vi "Inputs.vi"(8 "error in (no error)":errorcluster, 11 "State in":T1={"State"=enum."Idle", "Start Time"=timestamp(0 s since 1904-01-01), "Configuration"={"Cycle Period"=0.0, "Bronkhorst M13"={"VISA resource name"="", "Simulated?"=FALSE}, "Flow Meter Type"="", "Bronkhorst M14"={"VISA resource name"="", "Simulated?"=FALSE}}, "Current Time"=timestamp(0 s since 1904-01-01), "First Iteration"=FALSE, "Data"={"Flow Meter Read(g/min)"=0.0, "Density"=0.0, "Temp (C)"=0.0}, "Process Name"="", "Log Started"=FALSE}) -> (0 "error out":errorcluster, 3 "State out":T1={"State"=enum."Idle", "Start Time"=timestamp(0 s since 1904-01-01), "Configuration"={"Cycle Period"=0.0, "Bronkhorst M13"={"VISA resource name"="", "Simulated?"=FALSE}, "Flow Meter Type"="", "Bronkhorst M14"={"VISA resource name"="", "Simulated?"=FALSE}}, "Current Time"=timestamp(0 s since 1904-01-01), "First Iteration"=FALSE, "Data"={"Flow Meter Read(g/min)"=0.0, "Density"=0.0, "Temp (C)"=0.0}, "Process Name"="", "Log Started"=FALSE})   [LabVIEW 2018, in "Flow Module.lvlib" / "Flow Module Engine.lvlib"]
uses:
  Flow Module Engine.lvlib
  State Cluster.ctl
  State Enum.ctl
  Feed Module/Controls/Flow Module Settings Cluster.ctl
  Mettler Toledo/Controls/Settings Cluster.ctl
  Tag VIs/Tag FGV Operation Enum.ctl
  Bronkhorst M13 Flow Meter/Bronkhorst M13 Flow Meter.lvlib
  Bronkhorst M14 Flow Meter/Bronkhorst M14 Flow Meter.lvlib
  Shared Variables/Dynamic Shared Variables.lvlib
  Flow Module.lvlib
  Mettler Toledo/Mettler Toledo.lvlib
panel:
  # "Flow Meter Settings"
  # "Flow Meter Settings"
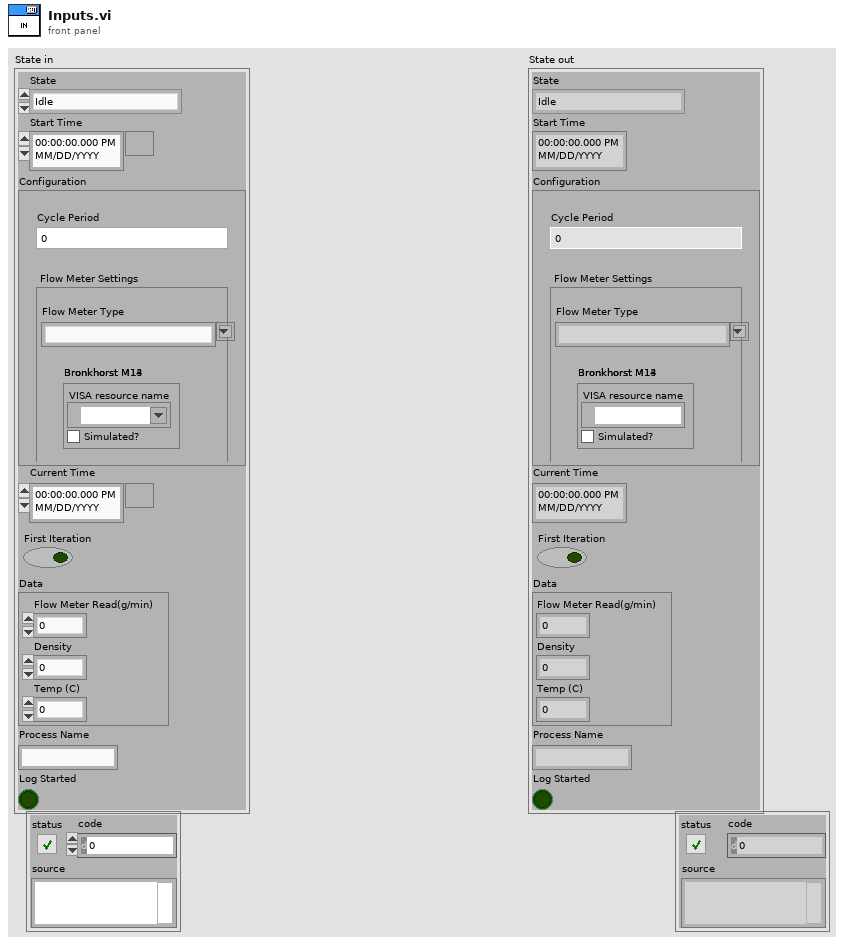
[diagram p1: front panel]
types:
  T1 = typedef "Flow Module.lvlib/Flow Module Engine.lvlib/State Cluster.ctl" = cluster{"State":T2, "Start Time":timestamp, "Configuration":T3, "Current Time":timestamp, "First Iteration":bool, "Data":cluster{"Flow Meter Read(g/min)":dbl, "Density":dbl, "Temp (C)":dbl}, "Process Name":string, "Log Started":bool}
  T2 = typedef "Flow Module.lvlib/Flow Module Engine.lvlib/State Enum.ctl" = enum16{"Measuring", "Idle"}
  T3 = typedef "Flow Module.lvlib/Flow Module Settings Cluster.ctl" = cluster{"Cycle Period":dbl, "Bronkhorst M13":T4, "Flow Meter Type":string, "Bronkhorst M14":T4}
  T4 = typedef "Mettler Toledo.lvlib/Settings Cluster.ctl" = cluster{"VISA resource name":refnum<visa-resource-name>, "Simulated?":bool}
  T5 = typedef "Tag FGV Operation Enum.ctl" = enum16{"Init", "Set Notification Queue", "Create Tag", "Commit", "Write Tag (Numeric)", "Write Tag (Boolean)", "Read All Tags", "Read One Tag", "Delete Tag Category", "Set Alarm Parameters (Numeric)", "Set Alarm Parameters (Boolean)", "Enable All Alarms", "Disable All Alarms", "Delete All Tags", "Read Alarms", "Ack Alarm", "Read Alarm Parameters (Numeric)", "Read Alarm Parameters (Boolean)"}
  T6 = typedef "Bronkhorst M13 Flow Meter.lvlib/Settings Cluster.ctl" = cluster{"VISA resource name":refnum<visa-resource-name>, "Simulated?":bool}
  T7 = typedef "Bronkhorst M14 Flow Meter.lvlib/Settings Cluster.ctl" = cluster{"VISA resource name":refnum<visa-resource-name>, "Simulated?":bool}
  T8 = typedef "Flow Module.lvlib/Tag Cluster.ctl" = cluster{"Flow Tag":string, "Input Disconnected":string, "Density Tag":string, "Temp Tag":string}
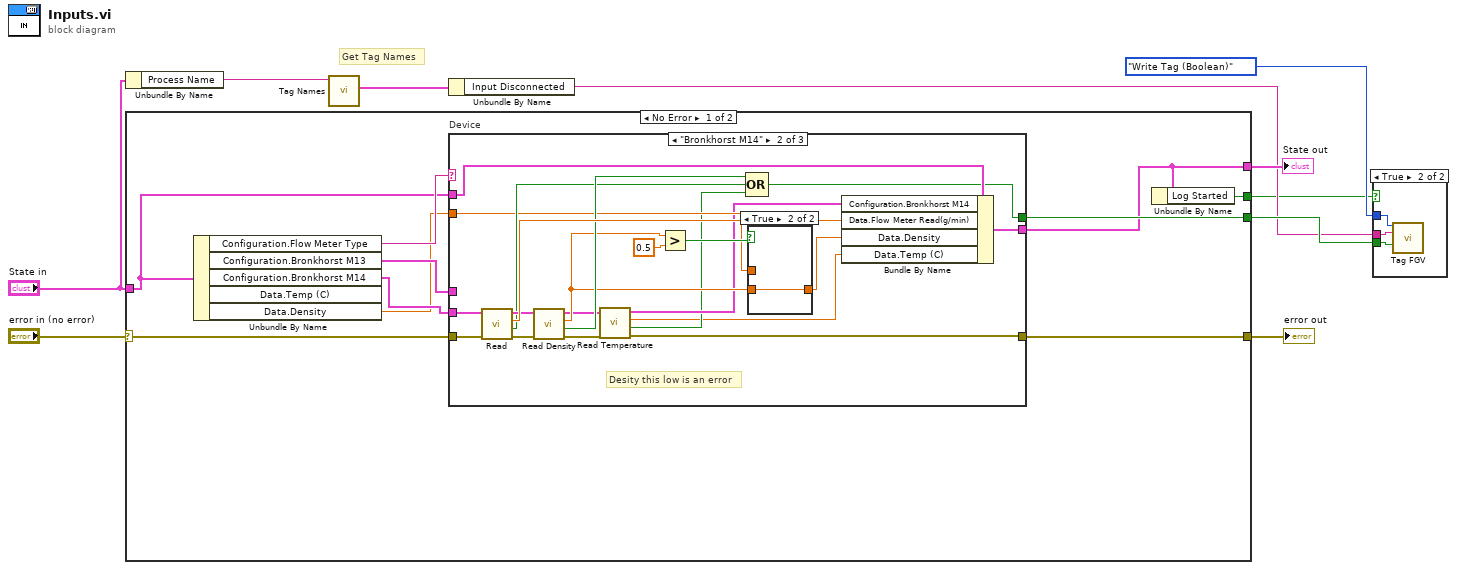
[diagram p0: block diagram]
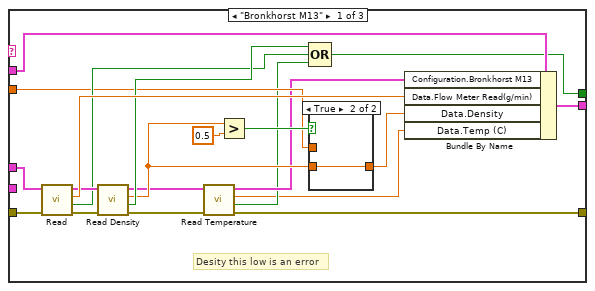
[diagram p3: hidden frame]
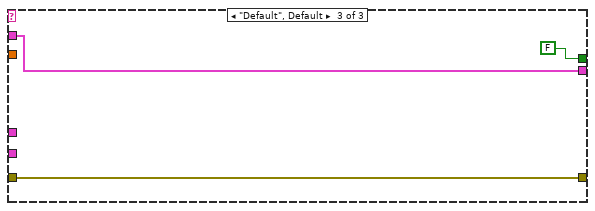
[diagram p6: hidden frame]
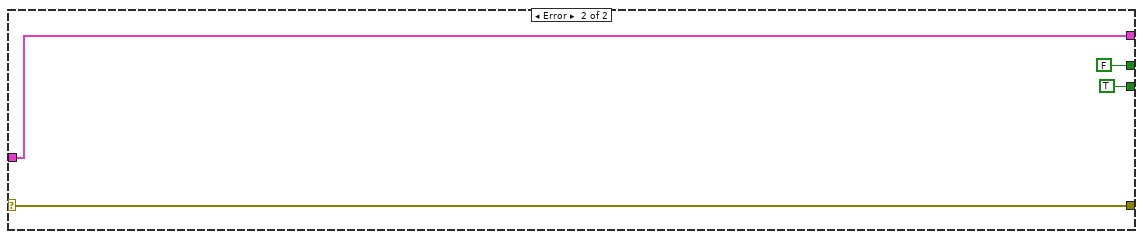
[diagram p7: hidden frame]
diagram:
  # "Get Tag Names"
  n1 = Unbundle By Name("State in") -> ("Process Name"=w7:string)
  n2 = case shown="No Error" "error in (no error)" {
    selector: "error in (no error)" -> [w18 w73]
    tunnel: [w17 w73] -> w8
    tunnel: "State in" -> [w16 w72]
    tunnel: [w12 w72] -> w9
    tunnel: [w14 TRUE ("Connection Error")] -> w4
    tunnel: [w11 FALSE ("Log Started")] -> w1
    frame No Error {
      n3 = Unbundle By Name(w16) -> ("Configuration.Flow Meter Type"=w20:string, "Configuration.Bronkhorst M13"=w19:T4, "Configuration.Bronkhorst M14"=w15:T4, "Data.Density"=w13:dbl)  [unwired: 1 out]
      n4 = case "Device" shown="\"Bronkhorst M14\"" w20 {
        tunnel: w16 -> [w39 w63 w69]
        tunnel: [w38 w62 w69] -> w12
        tunnel: w19 -> [w40 _ _]
        tunnel: w18 -> [w41 w64 w68]
        tunnel: [w25 w46 w68] -> w17
        tunnel: w13 -> [w27 w51 _]
        tunnel: w15 -> [_ w50 _]
        tunnel: [w34 w58 FALSE ("Connection Error")] -> w14
        frame "Bronkhorst M13" {
          # "Desity this low is an error"
          n5 = call "Read.vi"("error in (no error)"=w41, "Bronkhorst Settings in"=w40) -> ("error out"=w35:errorcluster, "Connection Error"=w32:bool, "flow"=w37:dbl, "Bronkhorst Settings out"=w36:T6)  [unwired: 6 in]
          n6 = call "Read Density.vi"("error in (no error)"=w35, "Bronkhorst Settings in"=w36) -> ("error out"=w26:errorcluster, "Connection Error"=w33:bool, "Density kg/m^3"=w28:sgl, "Bronkhorst Settings out"=w24:T6)  [unwired: 6 in]
          n7 = call "Read Temperature.vi"("error in (no error)"=w26, "Bronkhorst Settings in"=w24) -> ("error out"=w25:errorcluster, "Connection Error"=w22:bool, "Temp (C)"=w21:sgl, "Bronkhorst Settings out"=w23:T6)  [unwired: 6 in]
          n8 = Greater?(x=w28, y=0.5) -> (0:w30:bool)
          n9 = Compound Arithmetic op=OR(w33, w32, w22) -> (w34:bool)
          n10 = case shown="True" w30 {
            tunnel: [w42 w43] -> w29
            tunnel: w28 -> [_ w43]
            tunnel: w27 -> [w42 _]
            frame False {
            }
            frame True {
            }
          }
          n11 = Bundle By Name(cluster=w39, "Configuration.Bronkhorst M13"=w23, "Data.Flow Meter Read(g/min)"=w37, "Data.Density"=w29, "Data.Temp (C)"=w21) -> (w38:T1)
        }
        frame "Bronkhorst M14" {
          # "Desity this low is an error"
          n12 = call "Read.vi"("error in (no error)"=w64, "Bronkhorst Settings in"=w50) -> ("error out"=w59:errorcluster, "Connection Error"=w56:bool, "flow"=w61:dbl, "Bronkhorst Settings out"=w60:T7)  [unwired: 6 in]
          n13 = call "Read Density.vi"("error in (no error)"=w59, "Bronkhorst Settings in"=w60) -> ("error out"=w48:errorcluster, "Connection Error"=w57:bool, "Density kg/m^3"=w52:sgl, "Bronkhorst Settings out"=w49:T6)  [unwired: 6 in]
          n14 = call "Read Temperature.vi"("error in (no error)"=w48, "Bronkhorst Settings in"=w49) -> ("error out"=w46:errorcluster, "Connection Error"=w45:bool, "Temp (C)"=w44:sgl, "Bronkhorst Settings out"=w47:T6)  [unwired: 6 in]
          n15 = Greater?(x=w52, y=0.5) -> (0:w54:bool)
          n16 = Compound Arithmetic op=OR(w57, w56, w45) -> (w58:bool)
          n17 = case shown="True" w54 {
            tunnel: [w65 w66] -> w53
            tunnel: w52 -> [_ w66]
            tunnel: w51 -> [w65 _]
            frame False {
            }
            frame True {
            }
          }
          n18 = Bundle By Name(cluster=w63, "Configuration.Bronkhorst M14"=w47, "Data.Flow Meter Read(g/min)"=w61, "Data.Density"=w53, "Data.Temp (C)"=w44) -> (w62:T1)
        }
        frame "Default", Default {
        }
      }
      n19 = Unbundle By Name(w12) -> ("Log Started"=w11:bool)
    }
    frame Error {
    }
  }
  "error out" <- w8
  "State out" <- w9
  n20 = call "Tag Names.vi"("Process Name"=w7) -> ("Flow Tags"=w5:T8)  [unwired: 8 in, 2 out]
  n21 = Unbundle By Name(w5) -> ("Input Disconnected"=w3:string)
  n22 = case shown="True" w1 {
    tunnel: w4 -> [_ w76]
    tunnel: w3 -> [_ w75]
    tunnel: Tag_FGV_Operation_Enum."Write Tag (Boolean)" ("Operation") -> [_ w74]
    frame False {
    }
    frame True {
      n23 = call "Tag FGV.vi"("Operation"=w74, "Tag Name"=w75, "Data"=w76) -> ()  [unwired: 5 in, 8 out]
    }
  }
